vi "Check Guest History.vi"(0 "File Data Manager in":refnum<class "File Data Manager.lvclass">, 5 "Rooms Manager GUID":string, 7 "Guest Contact Number":string, 11 "error in (no error)":errorcluster) -> (4 "File Data Manager out":refnum<class "File Data Manager.lvclass">, 15 "error out":errorcluster)   [LabVIEW 2023, in "File Data Manager.lvlib" / "File Data Manager.lvclass"]
uses:
  File Data Manager.lvclass
  <vilib>/ActorFramework/Actor/Actor.lvclass/Actor.ctl
  File Data Manager.lvclass/File Data Manager.ctl
  Interfaces/Incoming Hotel Management Tool Model Interface Messages/Update Guest Name Msg/Update Guest Name Msg.lvclass/Update Guest Name Msg.ctl
  <vilib>/ActorFramework/Message Enqueuer/Message Enqueuer.lvclass/Message Enqueuer.ctl
  <vilib>/ActorFramework/Message Enqueuer/Enqueue.vi
  Interfaces/Incoming Hotel Management Tool Model Interface Messages/Update Guest Name Msg/Update Guest Name Msg.lvclass
  <vilib>/ActorFramework/Message Priority Queue/Priority Enqueue.vi
  <vilib>/ActorFramework/Actor/Actor.lvclass
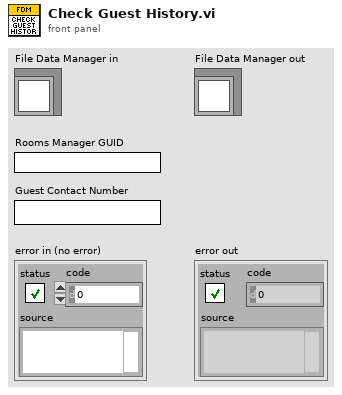
[diagram p1: front panel]
types:
  T1 = typedef "Central Data Manager.lvlib/Central Data Manager.lvclass/Guest Details.ctl" = cluster{"Contact Number":string, "Primary Guest Name":string}
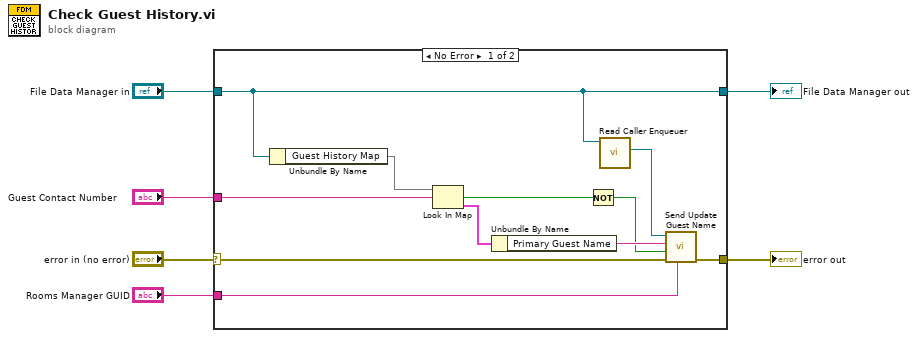
[diagram p0: block diagram]
diagram:
  n1 = case shown="No Error" "error in (no error)" {
    selector: "error in (no error)" -> [w17 w18]
    tunnel: [w16 w18] -> w5
    tunnel: "Rooms Manager GUID" -> [w15 _]
    tunnel: "File Data Manager in" -> [w7 w19]
    tunnel: "Guest Contact Number" -> [w12 _]
    tunnel: [w7 w19] -> w1
    frame No Error {
      n2 = Unbundle By Name(w7) -> ("Guest History Map"=w13:map{string, T1})
      n3 = Look In Map(map=w13, key=w12) -> (key not found?=w9:bool, value=w11:T1)  [unwired: 1 in]
      n4 = Unbundle By Name(w11) -> ("Primary Guest Name"=w10:string)
      n5 = Not(x=w9) -> (.not. x?=w8:bool)
      n6 = call <vilib>:"Read Caller Enqueuer.vi"("Actor"=w7) -> ("Caller Enqueuer"=w14:refnum<class "Message Enqueuer.lvclass">)  [unwired: 10 in]
      n7 = call "Send Update Guest Name.vi"("Rooms Manager GUID"=w15, "error in (no error)"=w17, "IsAvailable"=w8, "Guest Name"=w10, "Message Enqueuer"=w14) -> ("error out"=w16:errorcluster)  [unwired: 5 in, 1 out]
    }
    frame Error {
    }
  }
  "error out" <- w5
  "File Data Manager out" <- w1
